vi "Run Post-Render Hook.vi"(7 "Data":refnum<class "Datum.lvclass">, 8 "Error In":errorcluster, 10 "Hooks":T1, 11 "Writer In":refnum<class "Writer.lvclass">) -> (0 "Error Out":errorcluster, 3 "Writer Out":refnum<class "Writer.lvclass">)   [LabVIEW 2018, in "Toolkit.lvlib"]
uses:
  Data/Datum/Datum.lvclass
  Writers/Writer/Writer.lvclass
  Type Definitions/Hooks.ctl
  Hooks/Render/Render/Process.lvclass
  Hooks/Render/Section/Section.lvclass
  Hooks/Render/Variable/Variable.lvclass
  Toolkit.lvlib
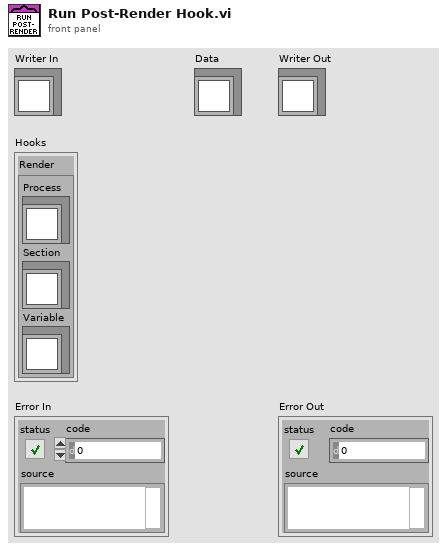
[diagram p1: front panel]
types:
  T1 = typedef "Toolkit.lvlib/Hooks.ctl" = cluster{"Render":cluster{"Process":refnum<class "Process.lvclass">, "Section":refnum<class "Section.lvclass">, "Variable":refnum<class "Variable.lvclass">}}
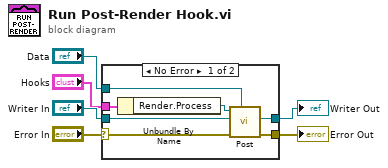
[diagram p0: block diagram]
diagram:
  n1 = case shown="No Error" "Error In" {
    selector: "Error In" -> [w7 w14]
    tunnel: "Data" -> [w12 _]
    tunnel: [w11 w15] -> w5
    tunnel: "Writer In" -> [w10 w15]
    tunnel: [w9 w14] -> w3
    tunnel: "Hooks" -> [w8 _]
    frame No Error {
      n2 = Unbundle By Name(w8) -> ("Render.Process"=w13:refnum<class "Process.lvclass">)
      n3 = call-dynamic "Post.vi"("Datum"=w12, "Error In"=w7, "Writer In"=w10, "Render In"=w13) -> ("Error Out"=w9:errorcluster, "Writer Out"=w11:refnum<class "Writer.lvclass">)  [unwired: 5 in, 1 out]
    }
    frame Error {
    }
  }
  "Writer Out" <- w5
  "Error Out" <- w3
